vi "FPGA_JKS_v1.vi"() -> ()   [LabVIEW 2014]
uses:
  <vilib>/LabVIEW Targets/FPGA/cRIO/shared/nicrio_ModuleControls/nicrio_cRIO-9237_ExcitationVoltageRing.ctl
  <vilib>/LabVIEW Targets/FPGA/cRIO/shared/nicrio_ModuleControls/nicrio_cRIO-9237_DataRatesRing.ctl
  <vilib>/rvi/Emulation/niFpgaGetClockAttributes.vi
  <vilib>/rvi/Emulation/niFpgaSctlEmulationGetInTimedLoop.vi
  <vilib>/rvi/Emulation/niFpgaEmulationReportErrorSimple.vi
  <vilib>/rvi/eio/common/nirviEmuTemplateMethod_errors.vi
  <vilib>/rvi/eio/common/nirviEmuTemplatePropertySet_noerrors.vi
  <vilib>/rvi/Emulation/niFpgaCriticalErrorInLSC.vi
  <vilib>/eio/EIONode/EIONode.xnode
  <vilib>/eio/EIOPropertyNode/EIOPropertyNode.xnode
  <vilib>/rvi/Analysis/measure/butterworth/XNode/niFpgaButterworthFilter.xnode
  <vilib>/rvi/eio/common/nirviEmuTemplatePropertyGet_errors.vi
  <vilib>/rvi/eio/common/nirviEmuTemplatePropertyGet_noerrors.vi
  <vilib>/rvi/eio/common/nirviEmuTemplatePropertySet_errors.vi
panel:
  out "Strain_unfiltered":fxp<+/-,24,3>
  out "Strain_filtered":fxp<+/-,24,3>
  in  "filter_coeff_strain":i32[](array[numeric])=[-898916953, 1957103773, 3888751]
  in  "Data Rate Strain Gauge":T1=1 items=["50.000 kS/s (NI 9237)"=1, "25.000 kS/s (NI 9237)"=2, "16.667 kS/s (NI 9237)"=3, "12.500 kS/s (NI 9237)"=4, "10.000 kS/s (NI 9237)"=5, "8.333 kS/s (NI 9237)"=6, "7.143 kS/s (NI 9237)"=7, "6.250 kS/s (NI 9237)"=8, "5.556 kS/s (NI 9237)"=9, "5.000 kS/s (NI 9237)"=10, "4.545 kS/s (NI 9237)"=11, "4.167 kS/s (NI 9237)"=12, "3.846 kS/s (NI 9237)"=13, "3.571 kS/s (NI 9237)"=14, "3.333 kS/s (NI 9237)"=15, "3.125 kS/s (NI 9237)"=16, "2.941 kS/s (NI 9237)"=17, "2.778 kS/s (NI 9237)"=18, "2.632 kS/s (NI 9237)"=19, "2.500 kS/s (NI 9237)"=20, "2.381 kS/s (NI 9237)"=21, "2.273 kS/s (NI 9237)"=22, "2.174 kS/s (NI 9237)"=23, "2.083 kS/s (NI 9237)"=24, "2.000 kS/s (NI 9237)"=25, "1.923 kS/s (NI 9237)"=26, "1.852 kS/s (NI 9237)"=27, "1.786 kS/s (NI 9237)"=28, "1.724 kS/s (NI 9237)"=29, "1.667 kS/s (NI 9237)"=30, "1.613 kS/s (NI 9237)"=31]
  in  "Excitation Voltage Strain Gauge":T2 items=["2.5 Volts", "3.3 Volts", "5.0 Volts", "10.0 Volts", "External Excitation"]
  in  "stop_inner_loop":bool
  out "FB_valves":fxp<+/-,20,9>[](array[numeric])=[0.001953125, 0.00439453125, 0.005859375]
  in  "filter_coeff_Hawe":i32[](array[numeric])=[-898916953, 1957103773, 3888751]
  in  "filter_coeff_Bosch":i32[](array[numeric])=[-898916953, 1957103773, 3888751]
  in  "filter_coeff_FB_PVG":i32[](array[numeric])=[-898916953, 1957103773, 3888751]
  out "actual_FPGA_filter_dt(uSec)":u32=20
  in  "FPGA_filter_dt(uSec)":u32=20
  in  "filter_coeff_Q":i32[](array[numeric])=[-898916953, 1957103773, 3888751]
  in  "filter_coeff_l_cyl":i32[](array[numeric])=[-898916953, 1957103773, 3888751]
  out "all_sensors":fxp<+/-,24,13>[](array[numeric])=[0.0107421875, 0.0078125, 0.04833984375, 1.791015625, 0.0107421875, 0.00830078125, 0.146484375, 5.01123046875]
  in  "filter_coeff_pressures":i32[](array[numeric])=[-898916953, 1957103773, 3888751]
  in  "reset_filters":bool
  in  "S_PVG":fxp<+/-,20,5>
  in  "stop_while_loop":bool
  in  "Sleep":bool
  in  "FPGA LED":bool
  in  "System Reset":bool
  out "Scan Clock":bool=TRUE
  out "Chassis Temperature":i16=129
  in  "S_Vickers":fxp<+/-,20,5>
  in  "S_Hawe":fxp<+/-,20,5>
  in  "S_Bosch":fxp<+/-,20,5>
  # "SETPOINT VALVES"
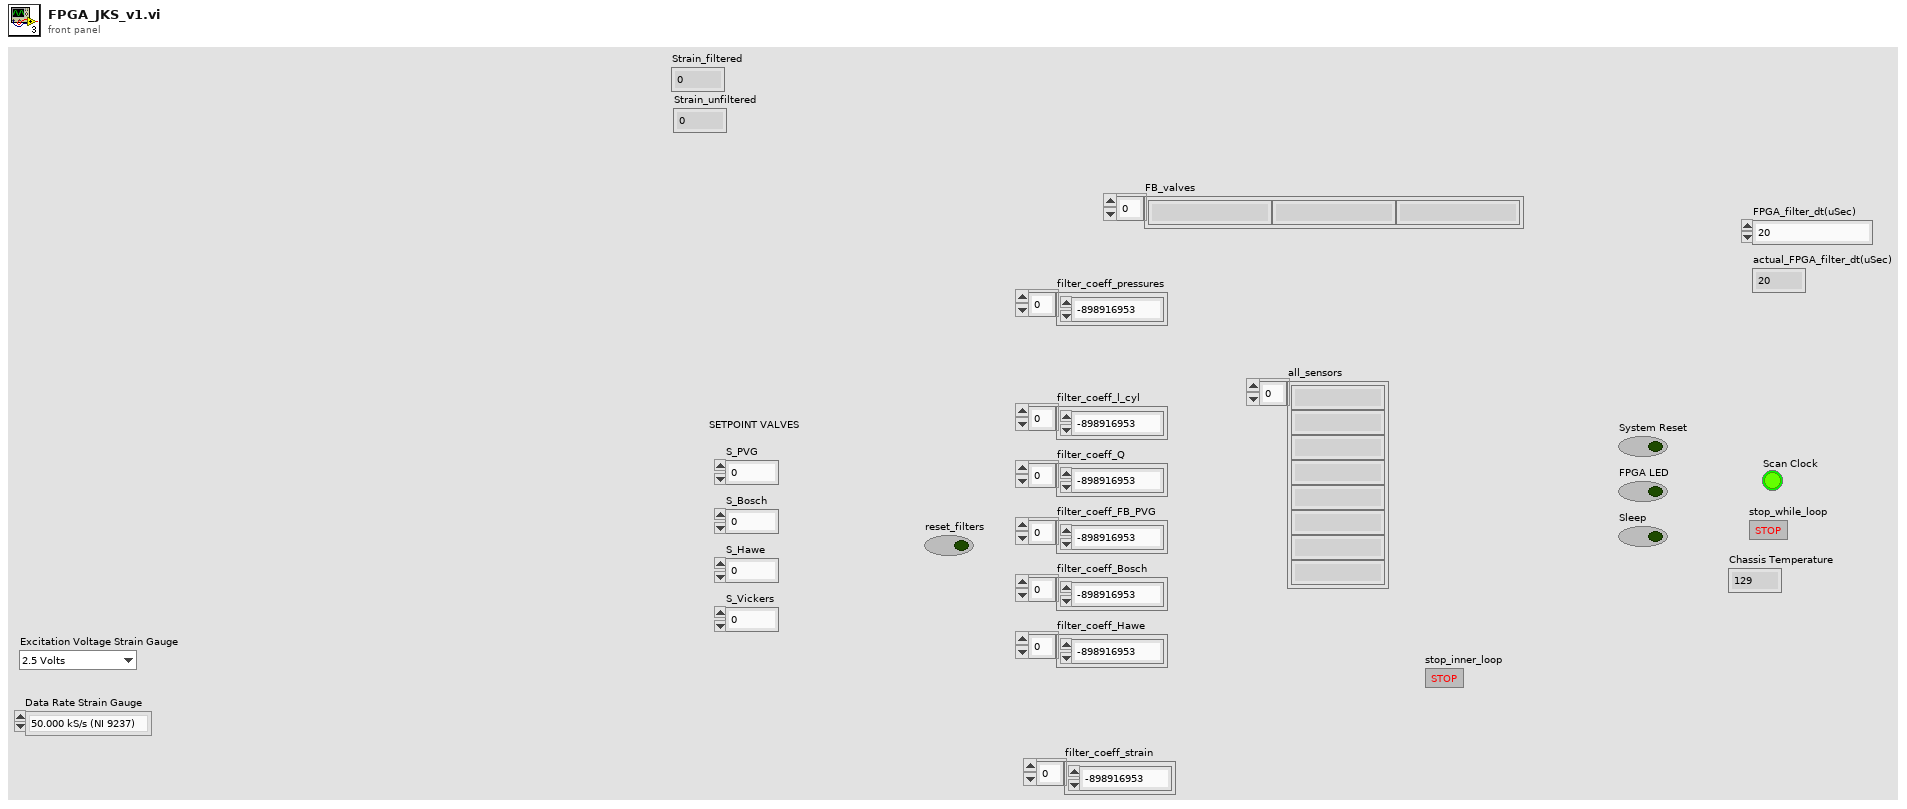
[diagram p1: front panel]
types:
  T1 = typedef "nicrio_cRIO-9237_DataRatesRing.ctl" = u8
  T2 = typedef "nicrio_cRIO-9237_ExcitationVoltageRing.ctl" = u8
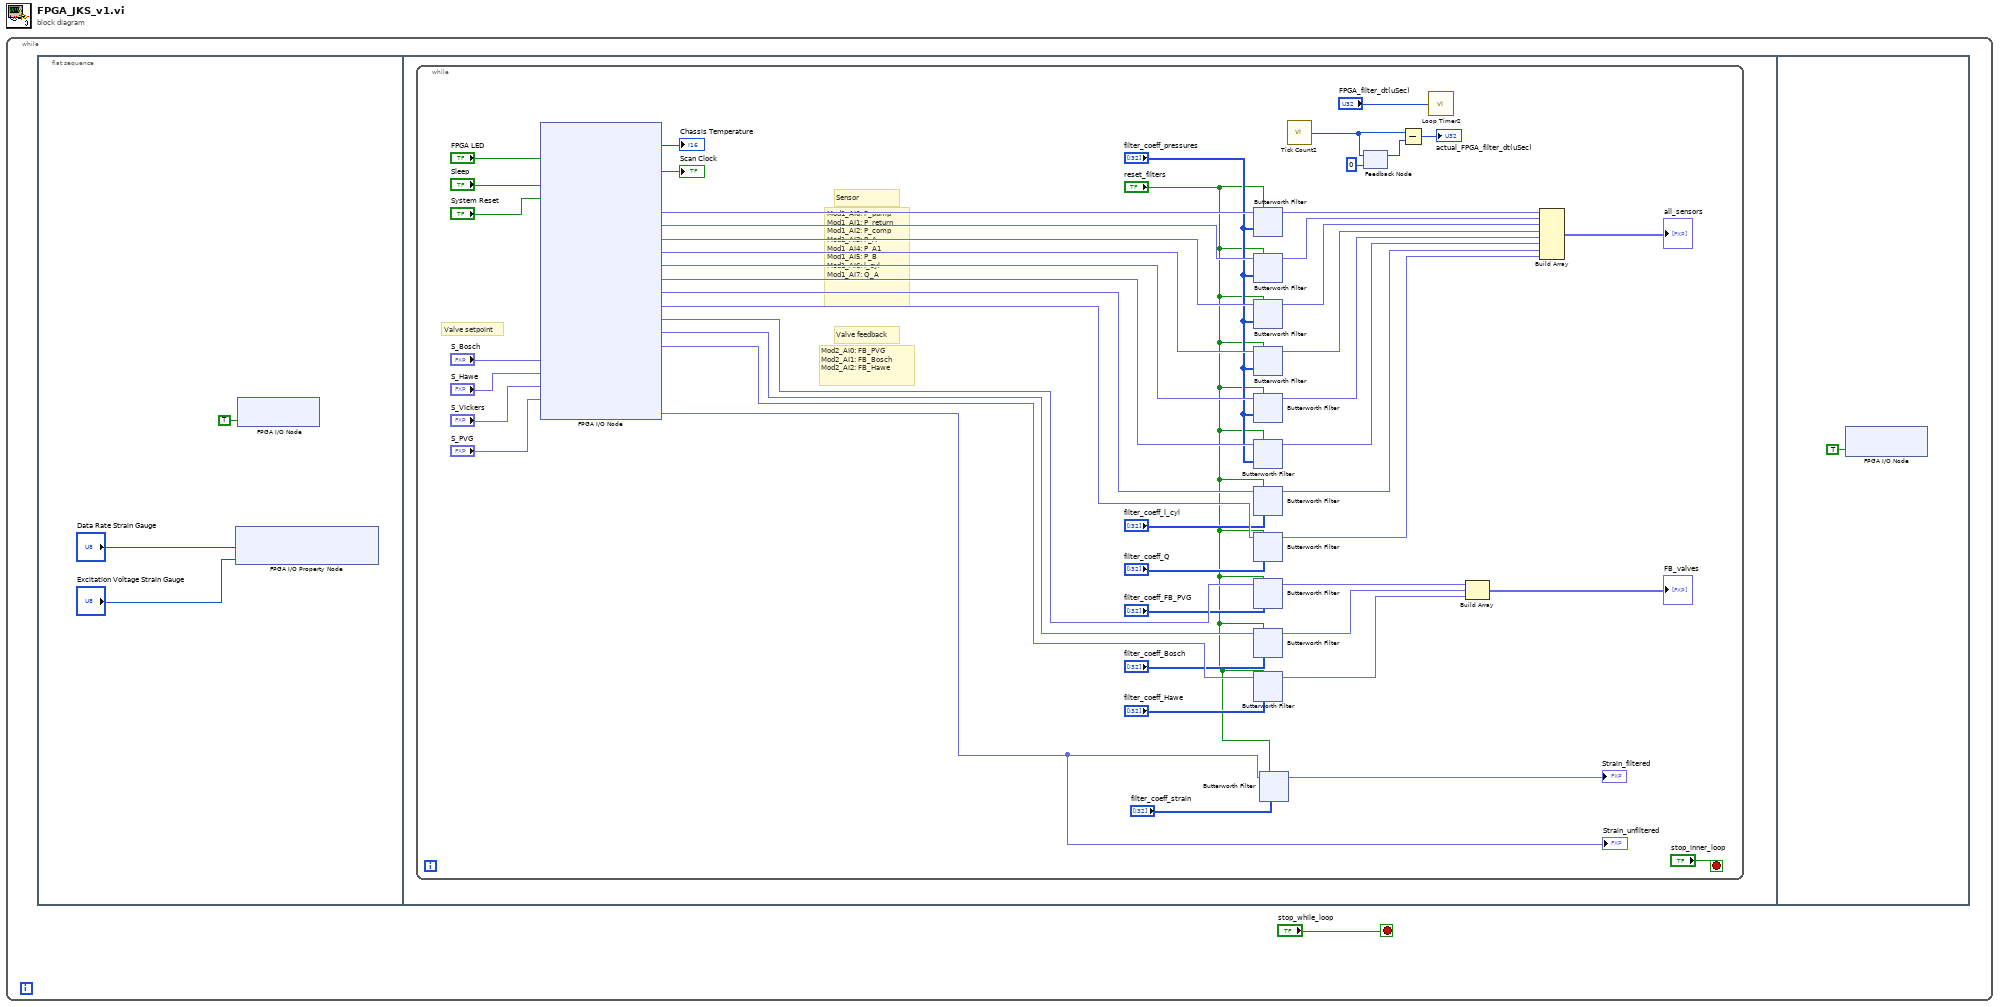
[diagram p0: block diagram]
diagram:
  n1 = while {
    stop <- "stop_while_loop" stop-if-true
    n2 = flat-sequence {
      frame #0 {
        n3 = xnode "FPGA I/O Property Node"("Data Rate"="Data Rate Strain Gauge", "Excitation Voltage"="Excitation Voltage Strain Gauge") -> ()  [unwired: 1 in, 1 out]
        n4 = xnode "FPGA I/O Node"("Mod4/Start"=TRUE) -> ()  [unwired: 1 in, 1 out]
      }
      frame #1 {
        n5 = while {
          stop <- "stop_inner_loop" stop-if-true
          # "Valve feedback"
          # "Sensor"
          # "Mod2_AI0: FB_PVG\nMod2_AI1: FB_Bosch\nMod2_AI2: FB_Hawe"
          # "Mod1_AI0: P_pump\nMod1_AI1: P_return\nMod1_AI2: P_comp\nMod1_AI3: P_A\nMod1_AI4: P_A1\nMod1_AI5: P_B\nMod1_AI6: l_cyl\nMod1_AI7: Q_A"
          # "Valve setpoint"
          n6 = xnode ("FPGA I/O Node")("FPGA LED"="FPGA LED", "Sleep"="Sleep", "System Reset"="System Reset", "Mod3/AO0"="S_Bosch", "Mod3/AO1"="S_Hawe", "Mod3/AO2"="S_Vickers", "Mod3/AO3"="S_PVG") -> ("Chassis Temperature"=→"Chassis Temperature":i16, "Scan Clock"=→"Scan Clock":bool, "Mod1/AI0"=w49:fxp<+/-,16,5>, "Mod1/AI1"=w50:fxp<+/-,16,5>, "Mod1/AI2"=w47:fxp<+/-,16,5>, "Mod1/AI3"=w44:fxp<+/-,16,5>, "Mod1/AI4"=w42:fxp<+/-,16,5>, "Mod1/AI5"=w41:fxp<+/-,16,5>, "Mod1/AI6"=w39:fxp<+/-,16,5>, "Mod1/AI7"=w38:fxp<+/-,16,5>, "Mod2/AI0"=w27:fxp<+/-,16,5>, "Mod2/AI1"=w26:fxp<+/-,16,5>, "Mod2/AI2"=w25:fxp<+/-,16,5>, "Mod4/AI0"=w5:fxp<+/-,24,-4>)  [unwired: 21 in, 21 out]
          "Strain_unfiltered" <- w5
          n7 = xnode "Butterworth Filter"("input data"=w49, "reset"="reset_filters", "scaled coefficients"="filter_coeff_pressures") -> ("output data"=w51:fxp<+/-,20,9>)
          n8 = xnode "Butterworth Filter"("input data"=w50, "reset"="reset_filters", "scaled coefficients"="filter_coeff_pressures") -> ("output data"=w48:fxp<+/-,20,9>)
          n9 = xnode "Butterworth Filter"("input data"=w47, "reset"="reset_filters", "scaled coefficients"="filter_coeff_pressures") -> ("output data"=w46:fxp<+/-,20,9>)
          n10 = xnode "Butterworth Filter"("input data"=w44, "reset"="reset_filters", "scaled coefficients"="filter_coeff_pressures") -> ("output data"=w45:fxp<+/-,20,9>)
          n11 = xnode "Butterworth Filter"("input data"=w42, "reset"="reset_filters", "scaled coefficients"="filter_coeff_pressures") -> ("output data"=w43:fxp<+/-,20,9>)
          n12 = xnode "Butterworth Filter"("input data"=w41, "reset"="reset_filters", "scaled coefficients"="filter_coeff_pressures") -> ("output data"=w35:fxp<+/-,20,9>)
          n13 = xnode "Butterworth Filter"("input data"=w39, "reset"="reset_filters", "scaled coefficients"="filter_coeff_l_cyl") -> ("output data"=w40:fxp<+/-,20,9>)
          n14 = xnode "Butterworth Filter"("input data"=w38, "reset"="reset_filters", "scaled coefficients"="filter_coeff_Q") -> ("output data"=w37:fxp<+/-,20,9>)
          n15 = xnode "Butterworth Filter"("input data"=w27, "reset"="reset_filters", "scaled coefficients"="filter_coeff_FB_PVG") -> ("output data"=w21:fxp<+/-,20,9>)
          n16 = xnode "Butterworth Filter"("input data"=w26, "reset"="reset_filters", "scaled coefficients"="filter_coeff_Bosch") -> ("output data"=w20:fxp<+/-,20,9>)
          n17 = xnode "Butterworth Filter"("input data"=w25, "reset"="reset_filters", "scaled coefficients"="filter_coeff_Hawe") -> ("output data"=w19:fxp<+/-,20,9>)
          n18 = xnode "Butterworth Filter"("input data"=w5, "reset"="reset_filters", "scaled coefficients"="filter_coeff_strain") -> ("output data"=→"Strain_filtered":fxp<+/-,28,0>)
          n19 = call "Tick Count2"() -> ("Tick Count(uSec)"=w30:u32)
          n20 = feedback #1(u32 0 ("Tick Count(uSec)")) -> (w28:u32)
          n21 = feedback-in #1(w30) -> ()
          n22 = Subtract(x=w30, y=w28) -> (x-y=→"actual_FPGA_filter_dt(uSec)":u32)
          n23 = call "Loop Timer2"("Count(uSec)"="FPGA_filter_dt(uSec)") -> ()  [unwired: 1 out]
          n24 = Build Array(w21, w20, w19) -> (→"FB_valves":fxp<+/-,20,9>[])
          n25 = Build Array(w51, w48, w46, w45, w43, w35, w40, w37) -> (→"all_sensors":fxp<+/-,20,9>[])
        }
      }
      frame #2 {
        n26 = xnode "FPGA I/O Node"("Mod4/Stop"=TRUE ("Mod4/Start")) -> ()  [unwired: 1 in, 1 out]
      }
    }
  }
